vi "trame_ana.vi"(10 "OKdém?":bool, 11 "Chaîne":string) -> (3 "Instruction":string)   [LabVIEW 2020]
doc: "Analyse la trame pour voir dans quel cas on bacsule"
uses:
  <vilib>/regexp/Match Regular Expression.xnode
panel:
  out "error out":errorcluster
  in  "errin":errorcluster
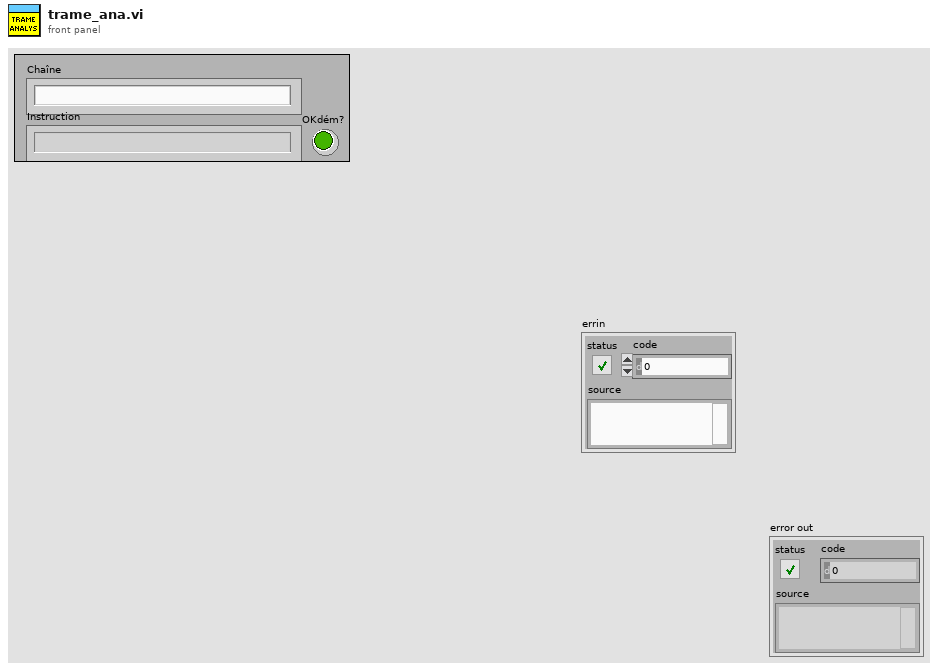
[diagram p1: front panel]
types:
  T1 = enum16{"open", "replace", "create", "open or create", "replace or create", "replace or create with confirmation"}
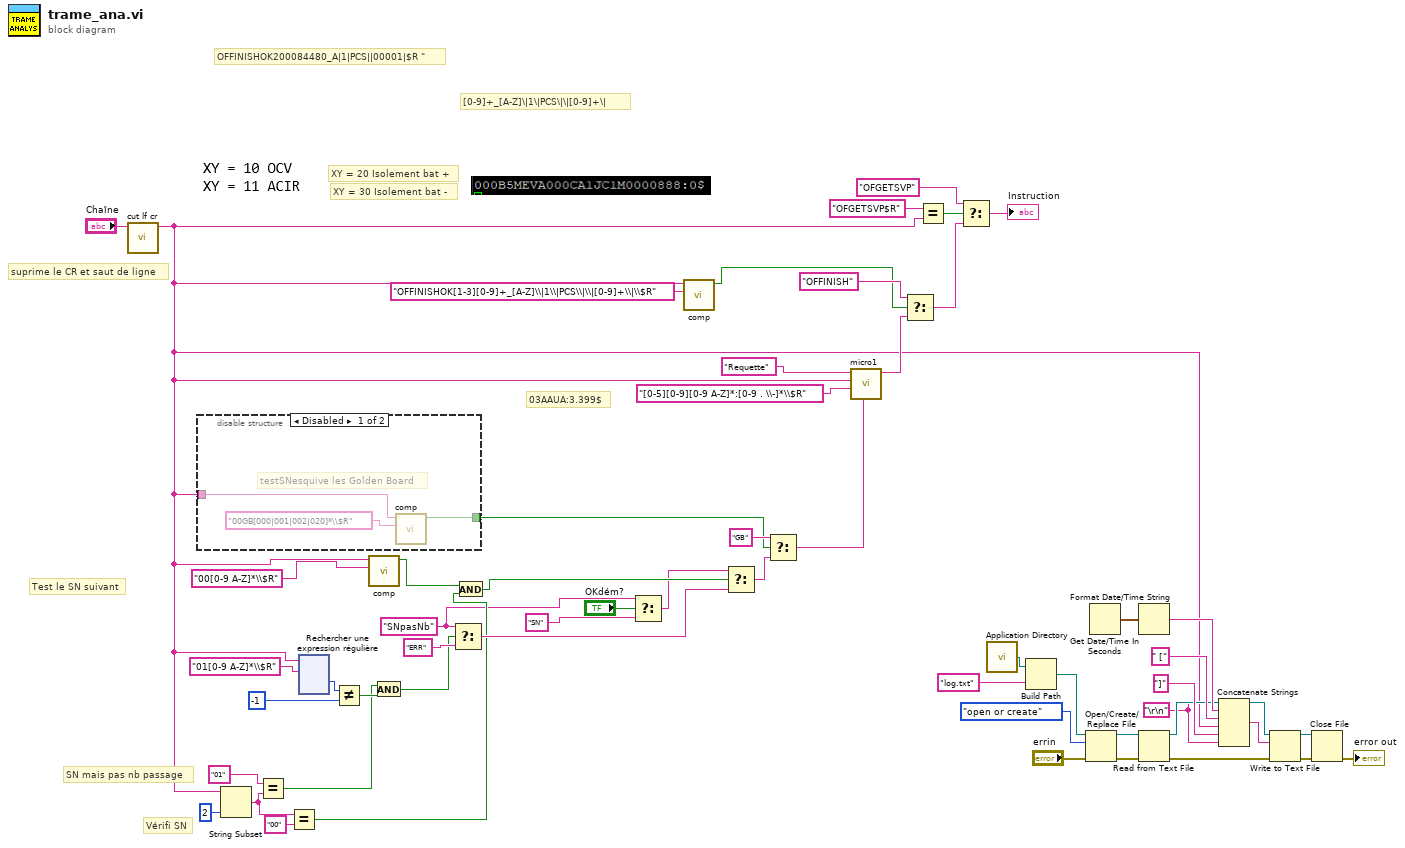
[diagram p0: block diagram]
diagram:
  w3 = "\r\n"
  w31 = "SNpasNb" ("cas vrai")
  # "[0-9]+_[A-Z]\\|1\\|PCS\\|\\|[0-9]+\\|"
  # "OFFINISHOK200084480_A|1|PCS||00001|$R \""
  # "Vérifi SN"
  # "SN mais pas nb passage"
  # "XY = 30 Isolement bat -"
  # "XY = 20 Isolement bat +"
  # "Test le SN suivant"
  # "suprime le CR et saut de ligne"
  # "03AAUA:3.399$"
  n1 = call "cut lf cr.vi"("strin"="Chaîne") -> ("strout"=w1:string)  [unwired: 10 in]
  n2 = disable-structure shown="Disabled" {
    disable-tunnel: [w58 _] -> w25
    disable-tunnel: w1 -> [w56 _]
    frame Disabled {
      # "testSNesquive les Golden Board"
      n3 = call "comp.vi"("expression régulière"="00GB[000|001|002|020]*\\$R", "strout"=w56) -> ("Boolean"=w58:bool)  [unwired: 9 in]
    }
    frame Enabled {
    }
  }
  n4 = String Subset ("Sous-ensemble d'une chaîne")(string=w1, length (rest)=2 ("longueur (reste)")) -> (substring=w39:string)  [unwired: 1 in]
  n5 = Equal? ("Égaux ?")(x="01", y=w39) -> (x = y?=w42:bool)
  n6 = Equal? ("Égaux ?")(x=w39, y="00") -> (x = y?=w37:bool)
  n7 = xnode "Rechercher une expression régulière"("chaîne en entrée"=w1, "expression régulière"="01[0-9 A-Z]*\\$R") -> ("offset après correspondance"=w46:i32)  [unwired: 4 in, 4 out]
  n8 = Not Equal? ("Différents ?")(x=w46, y=-1) -> (x != y?=w45:bool)
  n9 = call "comp.vi"("expression régulière"="00[0-9 A-Z]*\\$R", "strout"=w1) -> ("Boolean"=w24:bool)  [unwired: 9 in]
  n10 = And(x=w42, y=w45) -> (x .and. y?=w41:bool)
  n11 = Select ("Sélectionner")(t=w31, s=w41, f="ERR" ("cas faux")) -> (s? t:f=w49:string)
  n12 = And(x=w24, y=w37) -> (x .and. y?=w40:bool)
  n13 = Select ("Sélectionner")(t=w31, s="OKdém?", f="SN") -> (s? t:f=w32:string)
  n14 = call "comp.vi"("expression régulière"="OFFINISHOK[1-3][0-9]+_[A-Z]\\|1\\|PCS\\|\\|[0-9]+\\|\\$R", "strout"=w1) -> ("Boolean"=w22:bool)  [unwired: 9 in]
  n15 = Select ("Sélectionner")(t=w32, s=w40, f=w49) -> (s? t:f=w27:string)
  n16 = Select ("Sélectionner")(t="GB" ("cas vrai"), s=w25, f=w27) -> (s? t:f=w28:string)
  n17 = call "micro1.vi"("flux in en entrée"=w28, "expression régulière"="[0-5][0-9][0-9 A-Z]*:[0-9 . \\-]*\\$R", "data in"=w1, "cmd"="Requette") -> ("flux in en sortie"=w36:string)  [unwired: 7 in]
  n18 = Select ("Sélectionner")(t="OFFINISH", s=w22, f=w36) -> (s? t:f=w55:string)
  n19 = Equal? ("Égaux ?")(x="OFGETSVP$R", y=w1) -> (x = y?=w52:bool)
  n20 = Select(t="OFGETSVP", s=w52, f=w55) -> (s? t:f=→"Instruction":string)
  n21 = call <vilib>:"Application Directory.vi"() -> ("Application Directory"=w19:path)
  n22 = Build Path ("Composer un chemin")(base path=w19, name or relative path="log.txt") -> (appended path=w18:path)
  n23 = Open/Create/Replace File(file path (use dialog)=w18, error in="errin", operation (0:open)=T1."open or create") -> (refnum out=w6:refnum<file>, error out=w7:errorcluster)  [unwired: 3 in, 1 out]
  n24 = Get Date/Time In Seconds() -> (seconds since 1Jan1904=w12:timestamp)
  n25 = Format Date/Time String(seconds (now)=w12) -> (date/time string=w11:string)  [unwired: 2 in]
  n26 = Read from Text File(file (use dialog)=w6, error in=w7) -> (refnum out=w5:refnum<file>, error out=w8:errorcluster)  [unwired: 2 in, 2 out]
  n27 = Concatenate Strings(w3, w11, " [" ("string"), w1, "]" ("string"), w3) -> (w4:string)
  n28 = Write to Text File(file (use dialog)=w5, text=w4, error in=w8) -> (refnum out=w13:refnum<file>, error out=w15:errorcluster)  [unwired: 1 in, 1 out]
  n29 = Close File(refnum=w13, error in=w15) -> (error out=→"error out":errorcluster)  [unwired: 1 out]
